vi "markers.vi"(7 "Read?":bool=TRUE, 11 "markers":T1[](array[typedef])) -> (3 "markers out":T1[](array[typedef]))   [LabVIEW 2020, in "Graph Extensions.lvlib"]
uses:
  Graph Extensions.lvlib
  controls/MarkerInfo.ctl
  controls/markerType.ctl
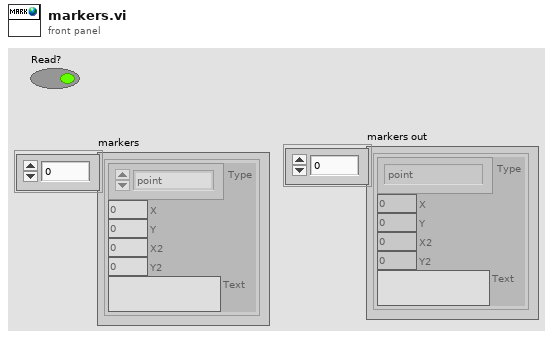
[diagram p1: front panel]
types:
  T1 = typedef "Graph Extensions.lvlib/MarkerInfo.ctl" = cluster{"Type":T2, "X":dbl, "Y":dbl, "X2":dbl, "Y2":dbl, "Text":string}
  T2 = typedef "Graph Extensions.lvlib/markerType.ctl" = enum16{"point", "arrow", "horiz", "vert", "vert range", "horiz range", "box"}
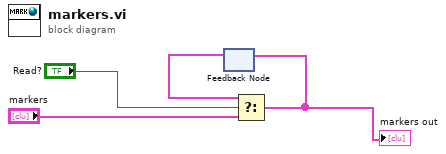
[diagram p0: block diagram]
diagram:
  n1 = feedback #1() -> (w3:T1[])  [unwired: 1 in]
  n2 = Select(t=w3, s="Read?", f="markers") -> (s? t:f=w1:T1[])
  "markers out" <- w1
  n3 = feedback-in #1(w1) -> ()
